vi "DefaultFromIni.vi"(8 "error in (no error)":errorcluster, 11 "MyPluginsBase in":refnum<class "Agilent_3458.lvclass">) -> (0 "error out":errorcluster, 3 "MyPluginsBase out":refnum<class "Agilent_3458.lvclass">)   [LabVIEW 2018, in "DigitizerPlugins.lvlib" / "Agilent_3458.lvclass"]
uses:
  Agilent_3458.lvclass
  F:/Program Files (x86)/National Instruments/LabVIEW 2018/user.lib/NIST/BaseClasses/BasePlugin_class/BasePlugin.lvclass
  <userlib>/NIST/BaseClasses/BasePlugin_class/BasePlugin.lvclass/BasePlugin.ctl
  Agilent_3458.lvclass/Agilent_3458.ctl
  <userlib>/NIST/BaseClasses/BasePlugin_class/Accessors/Read PluginIniFilePath.vi
  Accessors/Write Function (0_ DC Voltage).vi
  DigitizerBaseClass/DigitizerBase.lvclass
  <vilib>/Utility/config.llb/NI_LVConfig.lvlib
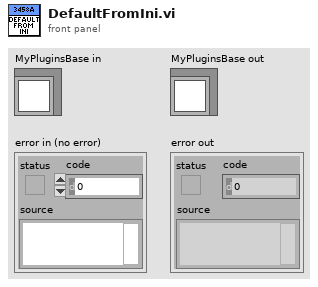
[diagram p1: front panel]
types:
  T1 = typedef "NI_LVConfig.lvlib/Config Data RefNum.ctl" = refnum<k1>
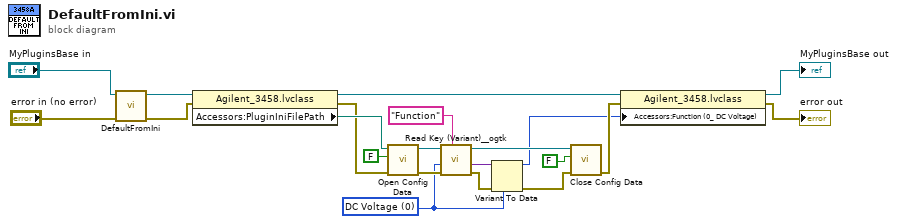
[diagram p0: block diagram]
diagram:
  w2 = u16 0 items=["DC Voltage", "AC Voltage", "AC + DC Voltage", "DC Current", "AC Current", "AC + DC Current", "2-Wire Resistance", "4-Wire Resistance", "Frequency", "Period", "Direct Sampling DC", "Direct Sampling AC", "Sub-Sampling DC", "Sub-Sampling AC"] ("Function (0: DC Voltage)")
  n1 = call-parent "DefaultFromIni.vi"("error in (no error)"="error in (no error)", "MyPluginsBase in"="MyPluginsBase in") -> ("error out"=w18:errorcluster, "MyPluginsBase out"=w21:refnum<class "Agilent_3458.lvclass">)  [unwired: 8 in]
  n2 = property class="Agilent_3458.lvclass"(reference=w21, error in=w18) -> (reference out=w10:refnum<class "Agilent_3458.lvclass">, error out=w16:errorcluster, "Accessors:PluginIniFilePath"=w17:path)
  n3 = call <vilib>:"Open Config Data.vi"("error in (no error)"=w16, "create file if necessary (T)"=FALSE, "configuration file path"=w17) -> ("error out"=w13:errorcluster, "refnum"=w14:T1)  [unwired: 6 in, 1 out]
  n4 = call <userlib>:"Read Key (Variant)__ogtk.vi"("section"="Function", "error in (no error)"=w13, "type"=w2, "refnum"=w14) -> ("error out"=w11:errorcluster, "key-value"=w12:variant, "refnum out"=w9:T1)  [unwired: 4 in, 1 out]
  n5 = Variant To Data(error in=w11, type=w2, Variant=w12) -> (data=w1:u16, error out=w8:errorcluster)
  n6 = call <vilib>:"Close Config Data.vi"("error in (no error)"=w8, "write file if changed (T)"=FALSE, "refnum"=w9) -> ("error out"=w5:errorcluster)  [unwired: 7 in, 1 out]
  n7 = property class="Agilent_3458.lvclass"(reference=w10, error in=w5, "Accessors:Function (0_ DC Voltage)"=w1) -> (reference out=→"MyPluginsBase out":refnum<class "Agilent_3458.lvclass">, error out=→"error out":errorcluster)
